vi "AddHeaderParams(DBL).vi"(0 "gfits refnum":T1, 11 "Error in":errorcluster, 13 "IntegerLine":T2(array[cluster])) -> (4 "dup gfits refnum":T1, 15 "Error out":errorcluster)   [LabVIEW 2019]
uses:
  gfitsio/gfitsio-refnum.ctl
  gfitsio/gfitsio.lvlib
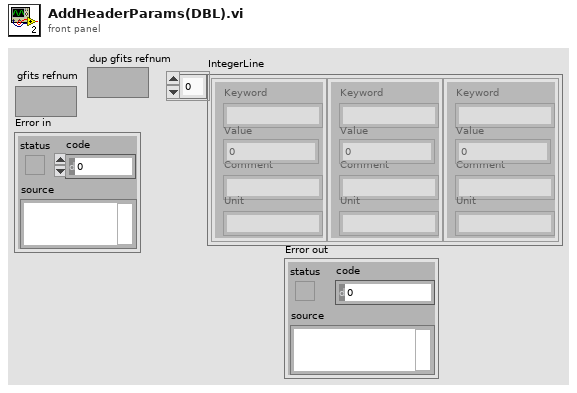
[diagram p1: front panel]
types:
  T1 = typedef "gfitsio.lvlib/gfitsio-refnum.ctl" = refnum<k1>
  T2 = cluster{"Keyword":string, "Value":dbl, "Comment":string, "Unit":string}[]
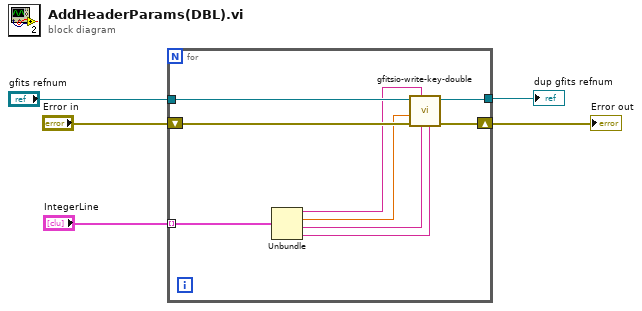
[diagram p0: block diagram]
diagram:
  n1 = for {
    tunnel: "gfits refnum" -> [w14]
    shift-right: [w12] -> w1
    shift-left: "Error in" -> [w13]
    tunnel: [w11] -> w2
    tunnel: "IntegerLine" -> [w10] mode=indexing
    n2 = Unbundle(w10) -> ("Keyword"=w9:string, "Value"=w8:dbl, "Comment"=w7:string, "Unit"=w6:string)
    n3 = call "gfitsio-write-key-double.vi"("units"=w6, "comment"=w7, "keyname"=w9, "error in (no error)"=w13, "value"=w8, "gfits refnum"=w14) -> ("error out"=w12:errorcluster, "dup gfits refnum"=w11:T1)  [unwired: 4 in]
  }
  "dup gfits refnum" <- w2
  "Error out" <- w1
